vi "Complex Vector x A (Optimized).vi"(2 "Matrix A":T1, 3 "Vector V'":cdb[](array[numeric])) -> (0 "error":i32, 1 "V' x A":cdb[](array[numeric]))   [LabVIEW 2017, in "NI_AALBase.lvlib"]
uses:
  <vilib>/Analysis/NI_AALBase.lvlib
  <vilib>/Analysis/Matrix/Datatypes/ComplexMatrix.ctl
  <resource>/lvanlys.dll
  <vilib>/Analysis/Matrix/NI_Matrix.lvlib
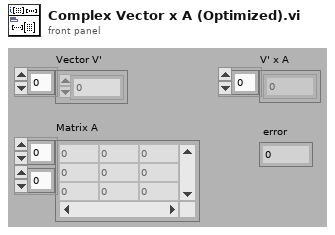
[diagram p1: front panel]
types:
  T1 = typedef "NI_Matrix.lvlib/ComplexMatrix.ctl" = cdb[][]
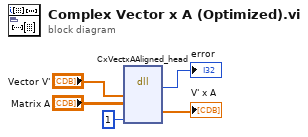
[diagram p0: block diagram]
diagram:
  n1 = dll-call lib="e:/builds/penguin/labview/branches/2017/dev/dist/resource/lvanlys.*" fn="CxVectxAAligned_head"("xHandle"="Vector V'", "aHandle"="Matrix A", "isAligned"=1) -> ("return type"=→"error":i32, "V' x A"=→"V' x A":cdb[])  [unwired: 7 in, 2 out]
